vi "imagesurfacelevel.vi"() -> ()   [LabVIEW 2015]
uses:
  ImageSurface.dll
  <vilib>/vision/NI_Vision_Development_Module.lvlib
panel:
  out "ImageSrc":T1(plugin-control)
  in  "Radius":i32=20
  in  "valueMin":i16
  in  "valueMax":i16=10000
  in  "SkipInvalidValue":bool=TRUE
  out "Return":i32
  out "ImageDst":T1(plugin-control)
  out "Point1Z":i16=1295
  out "Point2Z":i16=1278
  out "Point3Z":i16=1345
  out "Alpha 2":dbl=0.09707686755683868
  out "Beta 2":dbl=-0.07680741008059666
  out "Gamma 2":dbl=1309.996631781547
  in  "方法选择":bool
  out "字符串":string="方法1"
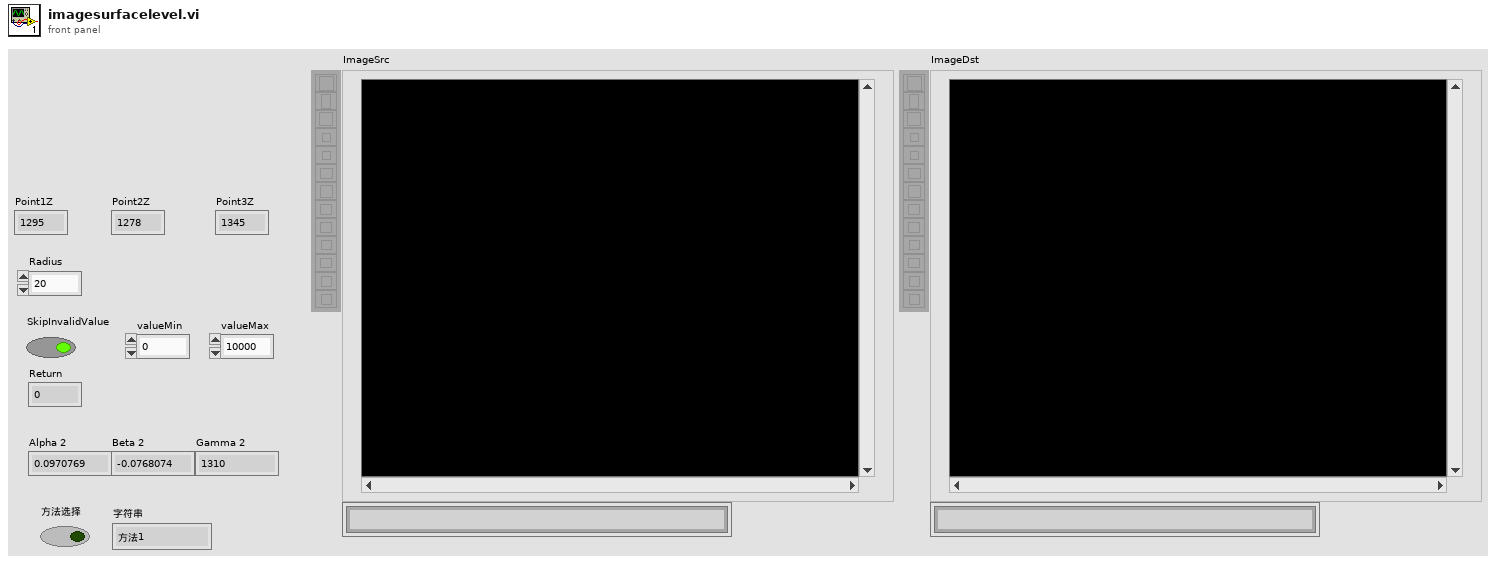
[diagram p1: front panel]
types:
  T1 = typedef "IMAQ Image.ctl" = refnum<image>
  T2 = typedef "Image Type" = u32
  T3 = typedef "ROI Descriptor" = cluster{"Global Rectangle":i32[], "Contours":cluster{"ID":enum32{"External", "Internal"}, "Type":u32, "Coordinates":i32[]}[]}
  T4 = cluster{"ID":enum32{"External", "Internal"}, "Type":u32, "Coordinates":i32[]}[]
  T5 = cluster{"ID":enum32{"External", "Internal"}, "Type":u32, "Coordinates":i32[]}
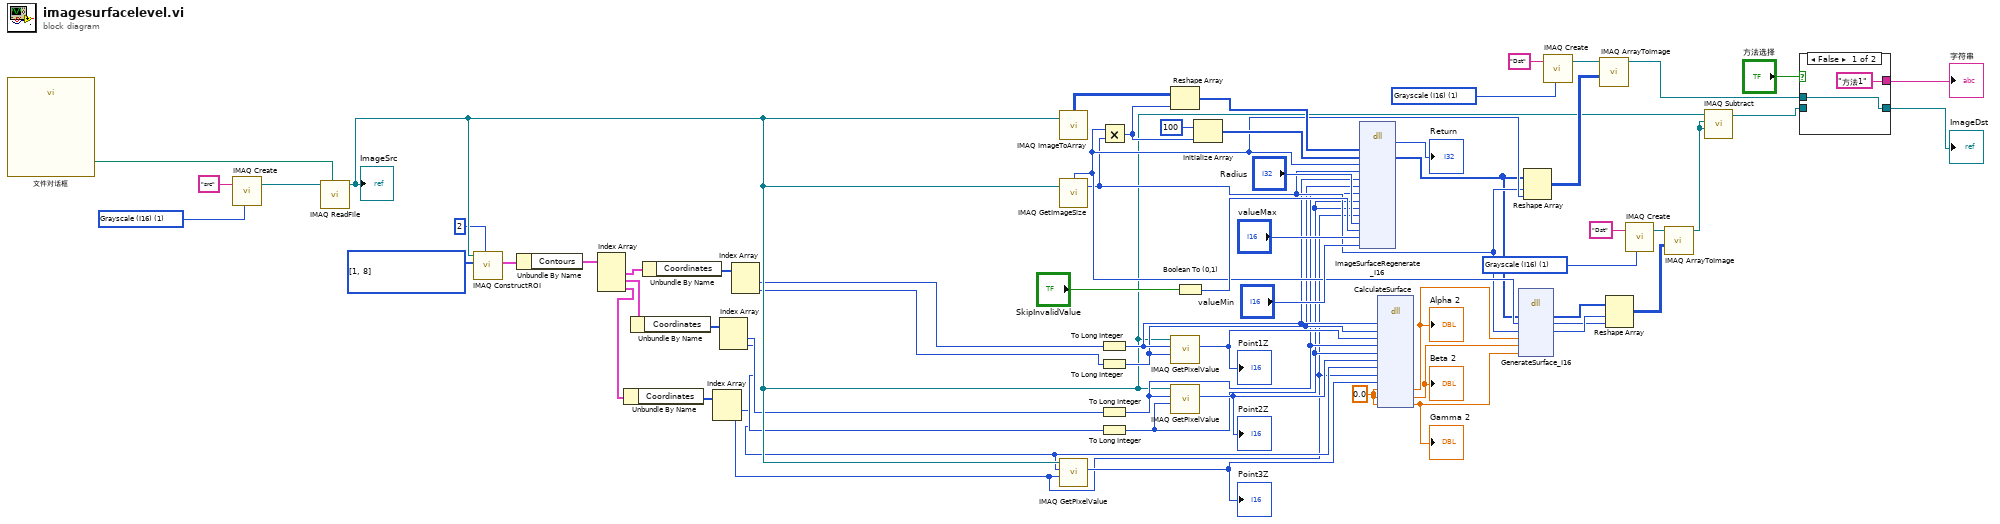
[diagram p0: block diagram]
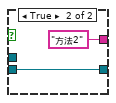
[diagram p2: hidden frame]
diagram:
  w15 = u32[] [1, 8] items=["No Selection", "Point", "Line", "Rectangle", "Oval", "Polygon", "Freehand Region", "Annulus", "Zoom", "Pan", "Broken Line", "Freehand Line", "Rotated Rectangle"] ("Tools")
  w24 = 0.0 ("Gamma")
  w33 = T2 1 items=["Grayscale (U8)", "Grayscale (I16)", "Grayscale (SGL)", "Complex (CSG)", "RGB (U32)", "HSL (U32)", "RGB (U64)", "Grayscale (U16)"] ("Image Type")
  w52 = T2 1 items=["Grayscale (U8)", "Grayscale (I16)", "Grayscale (SGL)", "Complex (CSG)", "RGB (U32)", "HSL (U32)", "RGB (U64)", "Grayscale (U16)"] ("Image Type")
  w62 = T2 1 items=["Grayscale (U8)", "Grayscale (I16)", "Grayscale (SGL)", "Complex (CSG)", "RGB (U32)", "HSL (U32)", "RGB (U64)", "Grayscale (U16)"] ("Image Type")
  n1 = call "文件对话框"() -> ("selected path"=w18:path)  [unwired: 12 in, 3 out]
  n2 = call "IMAQ Create"("Image Name"="src", "Image Type"=w62) -> ("New Image"=w61:T1)  [unwired: 3 in, 1 out]
  n3 = call "IMAQ ReadFile"("File Path"=w18, "Image"=w61) -> ("Image Out"=w17:T1)  [unwired: 5 in, 4 out]
  "ImageSrc" <- w17
  n4 = call "IMAQ ConstructROI"("Window Number (-1...15)"=2, "Tools"=w15, "Image"=w17) -> ("ROI Descriptor Out"=w14:T3)  [unwired: 5 in, 3 out]
  n5 = Unbundle By Name(w14) -> ("Contours"=w13:T4)
  n6 = Index Array(array=w13) -> (element #1=w12:T5, element #2=w6:T5, element #3=w5:T5)  [unwired: 3 in]
  n7 = Unbundle By Name(w5) -> ("Coordinates"=w7:i32[])
  n8 = Unbundle By Name(w6) -> ("Coordinates"=w8:i32[])
  n9 = Unbundle By Name(w12) -> ("Coordinates"=w11:i32[])
  n10 = Index Array(array=w7) -> (element #1=w2:i32, element #2=w1:i32)  [unwired: 2 in]
  n11 = Index Array(array=w8) -> (element #1=w4:i32, element #2=w3:i32)  [unwired: 2 in]
  n12 = Index Array(array=w11) -> (element #1=w10:i32, element #2=w9:i32)  [unwired: 2 in]
  n13 = call "IMAQ ImageToArray"("Image"=w17) -> ("Image Pixels (U8)"=w60:u8[][])  [unwired: 3 in, 4 out]
  n14 = call "IMAQ GetImageSize"("Image"=w17) -> ("Y Resolution"=w38:i32, "X Resolution"=w39:i32)  [unwired: 3 in, 1 out]
  n15 = call "IMAQ GetPixelValue"("Image"=w17, "X Coordinate"=w2, "Y Coordinate"=w1) -> ("Pixel Value (I16)"=w46:i16)  [unwired: 3 in, 4 out]
  "Point3Z" <- w46
  n16 = Multiply(x=w39, y=w38) -> (x*y=w49:i32)
  n17 = To Long Integer(number=w10) -> (32bit integer=w28:i32)
  n18 = To Long Integer(number=w9) -> (32bit integer=w27:i32)
  n19 = To Long Integer(number=w4) -> (32bit integer=w26:i32)
  n20 = To Long Integer(number=w3) -> (32bit integer=w25:i32)
  n21 = Reshape Array(w60, w49) -> (w55:u8[])
  n22 = call "IMAQ GetPixelValue"("Image"=w17, "X Coordinate"=w28, "Y Coordinate"=w27) -> ("Pixel Value (I16)"=w44:i16)  [unwired: 3 in, 4 out]
  "Point1Z" <- w44
  n23 = call "IMAQ GetPixelValue"("Image"=w17, "X Coordinate"=w26, "Y Coordinate"=w25) -> ("Pixel Value (I16)"=w45:i16)  [unwired: 3 in, 4 out]
  "Point2Z" <- w45
  n24 = Boolean To (0,1)(Boolean="SkipInvalidValue") -> (0, 1=w58:i16)
  n25 = Initialize Array(i16 100 ("元素"), w49) -> (w47:i16[])
  n26 = dll-call lib="PTH2¥abs Déæ é¡¹ç®æä»¶wnc LABVIEW2015\nåç»åRA01-AxxonSoftware WNC 20210806æºç -æå¨ä¸ä¼ æ¿åæµéçº¿æ¿..." fn="ImageSurfaceRegenerate_I16"("imageSrc"=w55, "imageDst"=w47, "nWidth"=w39, "nHeight"=w38, "nPoint1_X"=w28, "nPoint1_Y"=w27, "nPoint2_X"=w26, "nPoint2_Y"=w25, "nPoint3_X"=w25, "nPoint3_Y"=w1, "nDiamondRadius"="Radius", "bSkipInvalidValue"=w58, "valueMax"="valueMax", "valueMin"="valueMin") -> ("Return"=→"Return":i32, "imageDst"=w37:i16[])  [unwired: 16 in, 2 out]
  n27 = dll-call lib="PTH2¥abs Déæ é¡¹ç®æä»¶wnc LABVIEW2015\nåç»åRA01-AxxonSoftware WNC 20210806æºç -æå¨ä¸ä¼ æ¿åæµéçº¿æ¿..." fn="CalculateSurface"("X1"=w28, "Y1"=w27, "Z1"=w44, "X2"=w26, "Y2"=w25, "Z2"=w45, "X3"=w2, "Y3"=w1, "Z3"=w46, "Alpha"=w24, "Beta"=w24, "Gamma"=w24) -> ("Alpha"=w42:dbl, "Beta"=w41:dbl, "Gamma"=w40:dbl)  [unwired: 13 in, 2 out]
  "Alpha 2" <- w42
  "Beta 2" <- w41
  "Gamma 2" <- w40
  n28 = dll-call lib="PTH2¥abs Déæ é¡¹ç®æä»¶wnc LABVIEW2015\nåç»åRA01-AxxonSoftware WNC 20210806æºç -æå¨ä¸ä¼ æ¿åæµéçº¿æ¿..." fn="GenerateSurface_I16"("imageDst"=w37, "nWidth"=w39, "nHeight"=w38, "Alpha"=w42, "Beta"=w41, "Gamma"=w40) -> ("imageDst"=w32:i16[], "nWidth"=w30:i32, "nHeight"=w31:i32)  [unwired: 7 in, 2 out]
  n29 = Reshape Array(w37, w38, w39) -> (w43:i16[][])
  n30 = call "IMAQ Create"("Image Name"="Dst", "Image Type"=w52) -> ("New Image"=w50:T1)  [unwired: 3 in, 1 out]
  n31 = call "IMAQ ArrayToImage"("Image Pixels (I16)"=w43, "Image"=w50) -> ("Image Out"=w22:T1)  [unwired: 8 in, 1 out]
  n32 = Reshape Array(w32, w31, w30) -> (w36:i16[][])
  n33 = call "IMAQ Create"("Image Name"="Dst", "Image Type"=w33) -> ("New Image"=w35:T1)  [unwired: 3 in, 1 out]
  n34 = call "IMAQ ArrayToImage"("Image Pixels (I16)"=w36, "Image"=w35) -> ("Image Out"=w29:T1)  [unwired: 8 in, 1 out]
  n35 = call "IMAQ Subtract"("Image Src A"=w17, "Image Dst"=w29, "Image Src B"=w29) -> ("Image Dst Out"=w23:T1)  [unwired: 4 in, 1 out]
  n36 = case shown="False" "方法选择" {
    tunnel: w23 -> [_ w67]
    tunnel: [w65 w67] -> w19
    tunnel: w22 -> [w65 _]
    tunnel: ["方法1" "方法2"] -> w20
    frame False {
    }
    frame True {
    }
  }
  "ImageDst" <- w19
  "字符串" <- w20
